vi "Apply Glyph Transform.vi"(8 "error in (no error)":errorcluster, 9 "Transform in":refnum<class "Transform.lvclass">, 10 "glyph ref in":i64, 11 "Drawer":refnum<class "Freetype Drawer.lvclass">) -> (0 "error out":errorcluster, 2 "glyph ref out":i64, 3 "Drawer Out":refnum<class "Freetype Drawer.lvclass">)   [LabVIEW 2023, in "Freetype Drawer.lvlib" / "Freetype Drawer.lvclass"]
uses:
  Freetype Drawer.lvclass
  Font Glyph Drawer Interface/Transform/Transform.lvclass
  <vilib>/Analysis/Matrix/Datatypes/RealMatrix.ctl
  Freetype Drawer.lvclass/Freetype Drawer.ctl
  <vilib>/Analysis/baseanly.llb/Real A x B.vi
  Freetype Drawer.lvlib
  Font Glyph Drawer Interface/Font Glyph Drawer Interface.lvlib
  <vilib>/Analysis/NI_AALBase.lvlib
  <vilib>/Analysis/Matrix/NI_Matrix.lvlib
panel:
  out "Matrix Out":T1
  out "A x B":T1
  out "Transform":T1
  out "Size":cluster{"width":sgl, "height":sgl}
  out "Box":T2
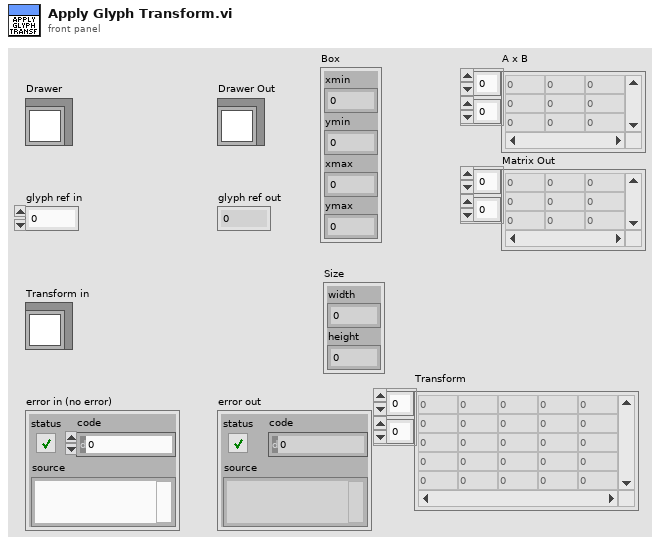
[diagram p1: front panel]
types:
  T1 = typedef "NI_Matrix.lvlib/RealMatrix.ctl" = dbl[][]
  T2 = cluster{"xmin":sgl, "ymin":sgl, "xmax":sgl, "ymax":sgl}
  T3 = typedef "Freetype Drawer.lvlib/Outline Glyph Rec.ctl" = cluster{"root":T4, "Outline":cluster{"n_contours":i16, "n_points":i16, "points ref":i64, "tags ref":i64, "contours ref":i64, "flags":i32}}
  T4 = typedef "Freetype Drawer.lvlib/Glyph Rec.ctl" = cluster{"library ref":i64, "class ref":i64, "format":i32, "advance":cluster{"x":i32, "y":i32}}
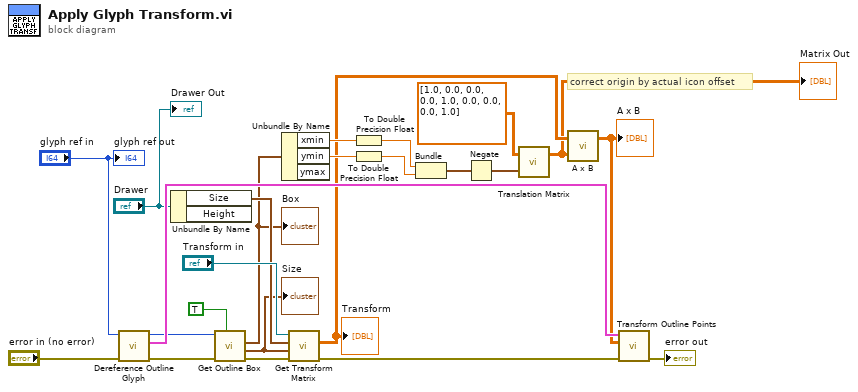
[diagram p0: block diagram]
diagram:
  # "correct origin by actual icon offset"
  n1 = call "Dereference Outline Glyph.vi"("error in (no error)"="error in (no error)", "glyph ref in"="glyph ref in") -> ("error out"=w14:errorcluster, "Outline Glyph Rec"=w18:T3, "glyph ref out"=w17:i64)  [unwired: 7 in]
  n2 = Unbundle By Name("Drawer") -> ("Size"=w11:cluster{"Width":u16, "Height":u16})  [unwired: 1 out]
  n3 = call "Get Outline Box.vi"("BBox (True)"=TRUE, "error in (no error)"=w14, "contour glyph ref"=w17) -> ("error out"=w15:errorcluster, "Size"=w5:cluster{"width":sgl, "height":sgl}, "Box"=w6:T2)  [unwired: 5 in, 1 out]
  "Box" <- w6
  "Size" <- w5
  n4 = Unbundle By Name(w6) -> ("xmin"=w20:sgl, "ymin"=w21:sgl)  [unwired: 1 out]
  n5 = call-dynamic "Get Transform Matrix.vi"("error in (no error)"=w15, "Glyph Size"=w5, "Canvas Size"=w11, "Transform in"="Transform in") -> ("error out"=w19:errorcluster, "Transform"=w3:T1)  [unwired: 5 in, 1 out]
  "Transform" <- w3
  n6 = To Double Precision Float(number=w20) -> (double precision float=w10:dbl)
  n7 = To Double Precision Float(number=w21) -> (double precision float=w9:dbl)
  n8 = Bundle(w10, w9) -> (w22:cluster{dbl, dbl})  [unwired: 1 in]
  n9 = Negate(x=w22) -> (-x=w23:cluster{dbl, dbl})
  n10 = call "Translation Matrix.vi"("Translation"=w23, "Matrix Type (2x3)"=T1 [[1.0, 0.0, 0.0], [0.0, 1.0, 0.0], [0.0, 0.0, 1.0]]) -> ("Matrix Out"=w1:T1)  [unwired: 1 in]
  "Matrix Out" <- w1
  n11 = call-poly <vilib>:"A x B.vi"("B"=w1, "A"=w3) -> ("A x B"=w2:T1)  [unwired: 1 out]
  "A x B" <- w2
  n12 = call "Transform Outline Points.vi"("error in (no error)"=w19, "2xN Matrix"=w2, "Outline Glyph Rec"=w18) -> ("error out"=→"error out":errorcluster)  [unwired: 7 in, 1 out]
  "glyph ref out" <- "glyph ref in"
  "Drawer Out" <- "Drawer"
